vi "BuildCameraCGI.vi"(2 "Acquire Params":T1={"fps"=10, "Compression"=30, "X"=320, "Y"=240, "Enable Color?"=TRUE, "Rotation"=enum."0"}, 3 "FPS?":bool, 4 "Get String":string) -> (1 "CGI String":string)   [LabVIEW 2017]
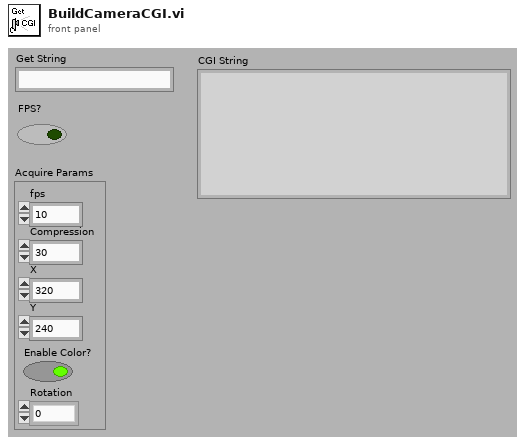
[diagram p1: front panel]
types:
  T1 = cluster{"fps":i32, "Compression":i32, "X":i32, "Y":i32, "Enable Color?":bool, "Rotation":enum16{"0", "90", "180", "270"}}
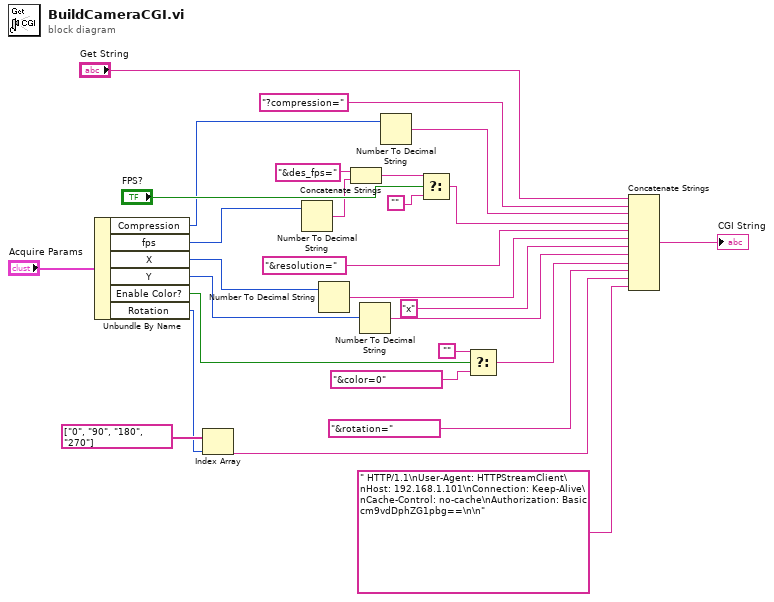
[diagram p0: block diagram]
diagram:
  n1 = Unbundle By Name("Acquire Params") -> ("Compression"=w6:i32, "fps"=w10:i32, "X"=w15:i32, "Y"=w16:i32, "Enable Color?"=w17:bool, "Rotation"=w18:enum16{"0", "90", "180", "270"})
  n2 = Index Array(array=string[] ["0", "90", "180", "270"], index=w18) -> (element=w2:string)
  n3 = Number To Decimal String(number=w10) -> (decimal integer string=w8:string)  [unwired: 1 in]
  n4 = Number To Decimal String(number=w15) -> (decimal integer string=w23:string)  [unwired: 1 in]
  n5 = Concatenate Strings("&des_fps=", w8) -> (w7:string)
  n6 = Number To Decimal String(number=w16) -> (decimal integer string=w25:string)  [unwired: 1 in]
  n7 = Number To Decimal String(number=w6) -> (decimal integer string=w21:string)  [unwired: 1 in]
  n8 = Select(t=w7, s="FPS?", f="") -> (s? t:f=w11:string)
  n9 = Select(t="", s=w17, f="&color=0") -> (s? t:f=w1:string)
  n10 = Concatenate Strings("Get String", "?compression=", w21, w11, "&resolution=", w23, "x", w25, w1, "&rotation=", w2, " HTTP/1.1\nUser-Agent: HTTPStreamClient\nHost: 192.168.1.101\nConnection: Keep-Alive\nCache-Control: no-cache\nAuthorization: Basic cm9vdDphZG1pbg==\n\n") -> (→"CGI String":string)
